vi "Copy Block Diagram.vi"(8 "error in (no error)":errorcluster, 10 "Dest In":refnum<vi>, 11 "Source In":refnum<vi>) -> (0 "error out":errorcluster, 2 "Dest":refnum<vi>, 3 "Source":refnum<vi>)   [LabVIEW 2020, in "FlexBlocks.lvlib"]
uses:
  FlexBlocks.lvlib
  <vilib>/Utility/miscctls.llb/LVPositionTypeDef.ctl
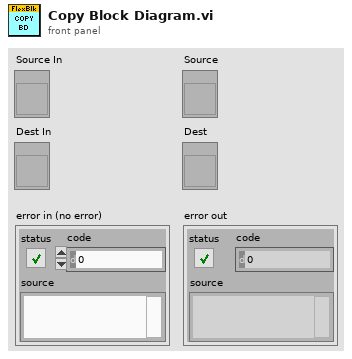
[diagram p1: front panel]
types:
  T1 = typedef "LVPositionTypeDef.ctl" = cluster{"Left":i32, "Top":i32}
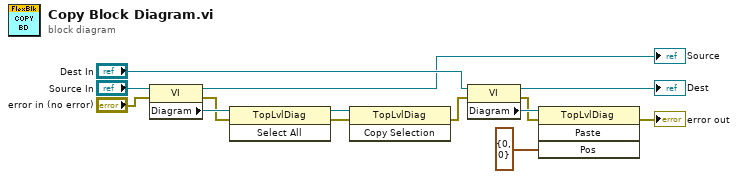
[diagram p0: block diagram]
diagram:
  n1 = property class="VI"(reference="Source In", error in="error in (no error)") -> (reference out=→"Source":refnum<vi>, error out=w12:errorcluster, "Diagram"=w14:refnum<vi>)
  n2 = invoke class="TopLvlDiag" method="Select All"(reference=w14, error in=w12) -> (reference out=w13:refnum<vi>, error out=w11:errorcluster)  [unwired: 1 in, 1 out]
  n3 = invoke class="TopLvlDiag" method="Copy Selection"(reference=w13, error in=w11) -> (error out=w4:errorcluster)  [unwired: 1 in, 2 out]
  n4 = property class="VI"(reference="Dest In", error in=w4) -> (reference out=→"Dest":refnum<vi>, error out=w9:errorcluster, "Diagram"=w10:refnum<vi>)
  n5 = invoke class="TopLvlDiag" method="Paste"(reference=w10, error in=w9, "Pos"=T1 {"Left"=0, "Top"=0} ("Position")) -> (error out=→"error out":errorcluster)  [unwired: 1 in, 3 out]
